vi "HFRR ADV v01.vi"() -> ()   [LabVIEW 2025] (continued)
                frame 81 {
                  n3062 = property on="Air Temperature  ( °C )" class="XYGraph (strict)"("Y Scale.Name Label.Text"=w4075) -> ()  [unwired: 2 in, 2 out]
                }
                frame 82 {
                  n3063 = local write "S 84"(w4076) -> ()
                }
                frame 83 {
                  n3064 = local write "S 85"(w4077) -> ()
                }
                frame 84 {
                  n3065 = local write "S 86"(w4078) -> ()
                }
                frame 85 {
                  n3066 = local write "S 87"(w4079) -> ()
                }
                frame 86 {
                  n3067 = local write "S 88"(w4080) -> ()
                }
                frame 87 {
                  n3068 = property on="FF Calibration g" class="WFGraph (strict)"("Y Scale.Name Label.Text"=w4081) -> ()  [unwired: 2 in, 2 out]
                }
                frame 88 {
                  n3069 = local write "S 90"(w4082) -> ()
                }
                frame 89 {
                  n3070 = local write "S 91"(w4083) -> ()
                }
                frame 90 {
                  n3071 = local write "S 92"(w4084) -> ()
                }
                frame 91 {
                  n3072 = local write "S 93"(w4085) -> ()
                }
                frame 92 {
                  n3073 = local write "S 94"(w4086) -> ()
                }
                frame 93 {
                  n3074 = local write "S 95"(w4087) -> ()
                }
                frame 94 {
                  n3075 = local write "S 96"(w4088) -> ()
                }
                frame 95 {
                  n3076 = local write "S 97"(w4089) -> ()
                }
                frame 96 {
                  n3077 = local write "S 98"(w4090) -> ()
                }
                frame 97 {
                  n3078 = local write "S 99"(w4091) -> ()
                }
                frame 98 {
                  n3079 = local write "S 100"(w4092) -> ()
                }
                frame 99 {
                  n3080 = local write "S 101"(w4093) -> ()
                }
                frame 100 {
                  n3081 = local write "S 102"(w4094) -> ()
                }
                frame 101 {
                  n3082 = local write "S 103"(w4095) -> ()
                }
                frame 102 {
                  n3083 = local write "S 104"(w4096) -> ()
                }
                frame 103 {
                  n3084 = local write "S 105"(w4097) -> ()
                }
                frame 104 {
                  n3085 = local write "S 106"(w4098) -> ()
                }
                frame 105 {
                }
                frame 106 {
                  n3086 = property on="OK Button 17" class="Bool (strict)"("Boolean Text.Text"=w4099) -> ()  [unwired: 2 in, 2 out]
                }
                frame 107 {
                  n3087 = property on="OK Button 16" class="Bool (strict)"("Boolean Text.Text"=w4100) -> ()  [unwired: 2 in, 2 out]
                }
                frame 108 {
                  n3088 = property on="TITTLE" class="Str"("Caption.Text"=w4101) -> ()  [unwired: 2 in, 2 out]
                }
                frame 109 {
                  "String 30" <- w4102
                }
                frame 110 {
                  n3089 = property on="Test Date" class="Str"("Caption.Text"=w4103) -> ()  [unwired: 2 in, 2 out]
                  "String 31" <- w4103
                }
                frame 111 {
                  n3090 = property on="Sample ID" class="Str"("Caption.Text"=w4104) -> ()  [unwired: 2 in, 2 out]
                  "String 32" <- w4104
                }
                frame 112 {
                  n3091 = property on="Tested by" class="Str"("Caption.Text"=w4105) -> ()  [unwired: 2 in, 2 out]
                  "String 33" <- w4105
                }
                frame 113 {
                  n3092 = property on="System Configured Printers 2" class="Arr (strict)"("Caption.Text"=w4106) -> ()  [unwired: 2 in, 2 out]
                }
                frame 114 {
                  n3093 = property on="Selected Printer" class="Str"("Caption.Text"=w4107) -> ()  [unwired: 2 in, 2 out]
                }
                frame 115 {
                  n3094 = property on="Select Printer 3" class="DigNum (strict)"("Caption.Text"=w4108) -> ()  [unwired: 2 in, 2 out]
                }
                frame 116 {
                  n3095 = property on="Print" class="Bool (strict)"("Boolean Text.Text"=w4109) -> ()  [unwired: 2 in, 2 out]
                }
                frame 117 {
                  "String 41" <- w4110
                }
                frame 118 {
                  n3096 = property on="tested by" class="Str"("Caption.Text"=w4111) -> ()  [unwired: 2 in, 2 out]
                }
                frame 119 {
                }
                frame 120 {
                  n3097 = property on="Export" class="Bool (strict)"("Boolean Text.Text"=w4112) -> ()  [unwired: 2 in, 2 out]
                }
                frame 121 {
                  n3098 = property on="TEMP INTERCEPT:" class="DigNum (strict)"("Caption.Text"=w4113) -> ()  [unwired: 2 in, 2 out]
                }
                frame 122 {
                  n3099 = property on="AIR TEMP INTERCEPT:" class="DigNum (strict)"("Caption.Text"=w4114) -> ()  [unwired: 2 in, 2 out]
                }
                frame 123 {
                  n3100 = property on="Select File Type" class="Enum (strict)"("Caption.Text"=w4115) -> ()  [unwired: 2 in, 2 out]
                }
                frame 124 {
                  n3101 = property on="s.NO" class="Str"("Caption.Text"=w4116) -> ()  [unwired: 2 in, 2 out]
                  "String 45" <- w4116
                }
                frame 125 {
                  n3102 = property on="trip1 8" class="Bool (strict)"("Boolean Text.Text"=w4117) -> ()  [unwired: 2 in, 2 out]
                }
                frame 126, Default {
                }
              }
            }
          }
          frame #1 {
            w4125 = TRUE ("Visible")
            n3103 = local read "S 91"() -> (w4142:string)
            n3104 = local read "S 90"() -> (w4141:string)
            n3105 = local read "S 88"() -> (w4140:string)
            n3106 = property on="File Path" class="Path"("Caption.Text"=w4141) -> ()  [unwired: 2 in, 2 out]
            n3107 = property on="SrvM CP" class="Bool (strict)"("Boolean Text.Text"=w4140) -> ()  [unwired: 2 in, 2 out]
            n3108 = local read "S 71"() -> (w4135:string)
            n3109 = local read "S 86"() -> (w4137:string)
            n3110 = local read "S 85"() -> (w4138:string)
            n3111 = local read "S 87"() -> (w4136:string)
            n3112 = local read "S 84"() -> (w4139:string)
            n3113 = local read "S 103"() -> (w4124:string)
            n3114 = local read "S 104"() -> (w4123:string)
            n3115 = property on="ENTER THE NEW PASSWORD" class="Str"("Caption.Text"=w4136) -> ()  [unwired: 2 in, 2 out]
            n3116 = property on="Password" class="Str"("Caption.Text"=w4138) -> ()  [unwired: 2 in, 2 out]
            n3117 = property on="ENTER CURRENT PASSWORD" class="Str"("Caption.Text"=w4137) -> ()  [unwired: 2 in, 2 out]
            n3118 = property on="EDIT" class="Bool (strict)"("Boolean Text.Text"=w4135) -> ()  [unwired: 2 in, 2 out]
            n3119 = property on="SAVE" class="Bool (strict)"("Boolean Text.Text"=w4139) -> ()  [unwired: 2 in, 2 out]
            n3120 = Build Array(w4124, w4123) -> (w4122:string[])
            n3121 = property on="Heater Button" class="Bool (strict)"("Strings [4]"=w4122) -> ()  [unwired: 2 in, 2 out]
            n3122 = property on="CH-HUMIDITY WET" class="DigNum (strict)"("Caption.Size to Text?"=w4125) -> ()  [unwired: 2 in, 2 out]
            n3123 = property on="CH-HUMIDITY DRY" class="DigNum (strict)"("Caption.Size to Text?"=w4125) -> ()  [unwired: 2 in, 2 out]
            n3124 = property on="CH-POWER -" class="DigNum (strict)"("Caption.Size to Text?"=w4125) -> ()  [unwired: 2 in, 2 out]
            n3125 = property on="CH-HEATER" class="DigNum (strict)"("Caption.Size to Text?"=w4125) -> ()  [unwired: 2 in, 2 out]
            n3126 = property on="CH-POWER +" class="DigNum (strict)"("Caption.Size to Text?"=w4125) -> ()  [unwired: 2 in, 2 out]
            n3127 = local read "S 92"() -> (w4134:string)
            n3128 = local read "S 93"() -> (w4133:string)
            n3129 = local read "S 105"() -> (w4120:string)
            n3130 = local read "S 106"() -> (w4119:string)
            n3131 = Build Array(w4134, w4133) -> ()  [unwired: 1 out]
            n3132 = Build Array(w4120, w4119) -> (w4121:string[])
            n3133 = local read "S 95"() -> (w4131:string)
            n3134 = local read "S 94"() -> (w4132:string)
            n3135 = local read "bs"() -> (w4147:string)
            n3136 = local read "as"() -> (w4148:string)
            n3137 = property on="Humidity" class="Bool (strict)"("Strings [4]"=w4121) -> ()  [unwired: 2 in, 2 out]
            n3138 = Concatenate Strings(w4147, "\r", w4148) -> ()  [unwired: 1 out]
            n3139 = property on="STROKE GAIN :" class="DigNum (strict)"("Caption.Text"=w4131) -> ()  [unwired: 2 in, 2 out]
            n3140 = property on="DISPLACEMENT :" class="DigNum (strict)"("Caption.Text"=w4132) -> ()  [unwired: 2 in, 2 out]
            n3141 = property on="Rh After" class="DigNum (strict)"("Caption.Size to Text?"=TRUE ("Caption.Size to Text")) -> ()  [unwired: 2 in, 2 out]
            n3142 = local read "S 48"() -> (w4171:string)
            n3143 = local read "S 50"() -> (w4169:string)
            n3144 = local read "S 51"() -> (w4168:string)
            n3145 = local read "S 49"() -> (w4170:string)
            n3146 = local read "S 52"() -> (w4167:string)
            n3147 = local read "as"() -> (w4152:string)
            n3148 = local read "bs"() -> (w4153:string)
            n3149 = local read "S 56"() -> (w4166:string)
            n3150 = local read "S 57"() -> (w4165:string)
            n3151 = local read "S 58"() -> (w4164:string)
            n3152 = local read "S 59"() -> (w4163:string)
            n3153 = property on="OPEN" class="Bool (strict)"("Boolean Text.Text"=w4167) -> ()  [unwired: 2 in, 2 out]
            n3154 = property on="OPEN 1" class="Bool (strict)"("Boolean Text.Text"=w4171) -> ()  [unwired: 2 in, 2 out]
            n3155 = property on="OPEN 2" class="Bool (strict)"("Boolean Text.Text"=w4170) -> ()  [unwired: 2 in, 2 out]
            n3156 = property on="OPEN 3" class="Bool (strict)"("Boolean Text.Text"=w4169) -> ()  [unwired: 2 in, 2 out]
            n3157 = property on="OPEN 4" class="Bool (strict)"("Boolean Text.Text"=w4168) -> ()  [unwired: 2 in, 2 out]
            n3158 = Concatenate Strings(w4153, "\r", w4152) -> ()  [unwired: 1 out]
            n3159 = local read "S 102"() -> (w4126:string)
            n3160 = property on="КОФ1" class="DigNum (strict)"("Caption.Text"=w4166) -> ()  [unwired: 2 in, 2 out]
            n3161 = local read "S 98"() -> (w4130:string)
            n3162 = local read "S 99"() -> (w4129:string)
            n3163 = local read "S 100"() -> (w4128:string)
            n3164 = local read "S 101"() -> (w4127:string)
            n3165 = property on="КОФ2" class="DigNum (strict)"("Caption.Text"=w4165) -> ()  [unwired: 2 in, 2 out]
            n3166 = property on="КОФ3" class="DigNum (strict)"("Caption.Text"=w4164) -> ()  [unwired: 2 in, 2 out]
            n3167 = property on="КОФ4" class="DigNum (strict)"("Caption.Text"=w4163) -> ()  [unwired: 2 in, 2 out]
            n3168 = local read "bs"() -> (w4151:string)
            n3169 = local read "as"() -> (w4150:string)
            n3170 = property on="CH-POWER +" class="DigNum (strict)"("Caption.Text"=w4130) -> ()  [unwired: 2 in, 2 out]
            n3171 = property on="CH-POWER -" class="DigNum (strict)"("Caption.Text"=w4129) -> ()  [unwired: 2 in, 2 out]
            n3172 = property on="CH-HEATER" class="DigNum (strict)"("Caption.Text"=w4128) -> ()  [unwired: 2 in, 2 out]
            n3173 = property on="CH-HUMIDITY DRY" class="DigNum (strict)"("Caption.Text"=w4127) -> ()  [unwired: 2 in, 2 out]
            n3174 = property on="CH-HUMIDITY WET" class="DigNum (strict)"("Caption.Text"=w4126) -> ()  [unwired: 2 in, 2 out]
            n3175 = local read "S 60"() -> (w4162:string)
            n3176 = local read "S 54"() -> (w4172:string)
            n3177 = Concatenate Strings(w4151, "\r", w4150) -> ()  [unwired: 1 out]
            n3178 = Concatenate Strings(w4172, w4162) -> ()  [unwired: 1 out]
            n3179 = local read "S 77"() -> (→"String 43":string)
            n3180 = local read "S 76"() -> (w4145:string)
            n3181 = local read "S 78"() -> (w4144:string)
            n3182 = local read "S 71"() -> (w4156:string)
            n3183 = local read "S 66"() -> (w4161:string)
            n3184 = local read "S 67"() -> (w4160:string)
            n3185 = local read "S 68"() -> (w4159:string)
            n3186 = local read "S 69"() -> (w4158:string)
            n3187 = local read "S 70"() -> (w4157:string)
            n3188 = property on="AIR TEMP" class="DigNum (strict)"("Caption.Text"=w4144) -> ()  [unwired: 2 in, 2 out]
            n3189 = property on="Set Strk" class="DigNum (strict)"("Caption.Text"=w4145) -> ()  [unwired: 2 in, 2 out]
            n3190 = property on="FRIC. FORCE :" class="DigNum (strict)"("Caption.Text"=w4161) -> ()  [unwired: 2 in, 2 out]
            n3191 = property on="TEMPERATURE :" class="DigNum (strict)"("Caption.Text"=w4160) -> ()  [unwired: 2 in, 2 out]
            n3192 = property on="SPEED OUT:" class="DigNum (strict)"("Caption.Text"=w4159) -> ()  [unwired: 2 in, 2 out]
            n3193 = property on="AIR TEMPERATURE :" class="DigNum (strict)"("Caption.Text"=w4158) -> ()  [unwired: 2 in, 2 out]
            n3194 = property on="HUMIDITY:" class="DigNum (strict)"("Caption.Text"=w4157) -> ()  [unwired: 2 in, 2 out]
            n3195 = property on="EDIT" class="Bool (strict)"("Boolean Text.Text"=w4156) -> ()  [unwired: 2 in, 2 out]
            n3196 = local read "S 79"() -> (w4143:string)
          }
          frame #2 {
          }
        }
        n3197 = local write "Lan flag"(10.0 ("Lan flag")) -> ()
      }
      frame Enabled {
      }
    }
    n3198 = Wait (ms)(milliseconds to wait=u32 2000) -> ()  [unwired: 1 out]
    n3199 = local read "Quit"() -> (w3945:bool)
  }
  n3200 = disable-structure shown="Disabled" {
    frame Disabled {
      n3201 = while {
        tunnel: [w4174] -> _
        i -> [w4174]
        stop <- w4173 continue-if-true
        n3202 = Wait (ms)(milliseconds to wait=u32 50) -> ()  [unwired: 1 out]
        n3203 = stacked-sequence {
          frame #0 {
            # "Controls Text color"
            # "Controls BG color"
            n3204 = property on="FILE" class="Str"("Text.Text Colors:Text Color"="SC  Text") -> ()  [unwired: 2 in, 2 out]
            n3205 = property on="Fuel Discription :" class="Str"("Text.Text Colors:Text Color"="SC  Text") -> ()  [unwired: 2 in, 2 out]
            n3206 = property on="tested by" class="Str"("Text.Text Colors:Text Color"="SC  Text") -> ()  [unwired: 2 in, 2 out]
            n3207 = property on="Remarks :" class="Str"("Text.Text Colors:Text Color"="SC  Text") -> ()  [unwired: 2 in, 2 out]
            n3208 = property class="DigNum (strict)"("Numeric Text.Text Colors:BG Color"="NC BG") -> ()  [unwired: 2 in, 2 out]
            n3209 = property class="DigNum (strict)"("Numeric Text.Text Colors:BG Color"="NC BG") -> ()  [unwired: 2 in, 2 out]
            n3210 = property class="DigNum (strict)"("Numeric Text.Text Colors:BG Color"="NC BG") -> ()  [unwired: 2 in, 2 out]
            n3211 = property class="DigNum (strict)"("Numeric Text.Text Colors:BG Color"="NC BG") -> ()  [unwired: 2 in, 2 out]
            n3212 = property class="DigNum (strict)"("Numeric Text.Text Colors:BG Color"="NC BG") -> ()  [unwired: 2 in, 2 out]
            n3213 = property class="DigNum (strict)"("Numeric Text.Text Colors:BG Color"="NC BG") -> ()  [unwired: 2 in, 2 out]
            n3214 = property class="DigNum (strict)"("Numeric Text.Text Colors:BG Color"="NC BG") -> ()  [unwired: 2 in, 2 out]
            n3215 = property class="DigNum (strict)"("Numeric Text.Text Colors:BG Color"="NC BG") -> ()  [unwired: 2 in, 2 out]
            n3216 = property class="DigNum (strict)"("Numeric Text.Text Colors:BG Color"="NC BG") -> ()  [unwired: 2 in, 2 out]
            n3217 = property class="DigNum (strict)"("Numeric Text.Text Colors:BG Color"="NC BG") -> ()  [unwired: 2 in, 2 out]
            n3218 = property class="DigNum (strict)"("Numeric Text.Text Colors:BG Color"="NC BG") -> ()  [unwired: 2 in, 2 out]
            n3219 = property class="DigNum (strict)"("Numeric Text.Text Colors:BG Color"="NC BG") -> ()  [unwired: 2 in, 2 out]
            n3220 = property on="FILE" class="Str"("Text.Text Colors:BG Color"="SC BG 3") -> ()  [unwired: 2 in, 2 out]
            n3221 = property on="Fuel Discription :" class="Str"("Text.Text Colors:BG Color"="SC BG 3") -> ()  [unwired: 2 in, 2 out]
            n3222 = property on="tested by" class="Str"("Text.Text Colors:BG Color"="SC BG 3") -> ()  [unwired: 2 in, 2 out]
            n3223 = property on="Remarks :" class="Str"("Text.Text Colors:BG Color"="SC BG 3") -> ()  [unwired: 2 in, 2 out]
            n3224 = property class="DigNum (strict)"("Numeric Text.Text Colors:Text Color"="NC Text") -> ()  [unwired: 2 in, 2 out]
            n3225 = property class="DigNum (strict)"("Numeric Text.Text Colors:Text Color"="NC Text") -> ()  [unwired: 2 in, 2 out]
            n3226 = property class="DigNum (strict)"("Numeric Text.Text Colors:Text Color"="NC Text") -> ()  [unwired: 2 in, 2 out]
            n3227 = property class="DigNum (strict)"("Numeric Text.Text Colors:Text Color"="NC Text") -> ()  [unwired: 2 in, 2 out]
            n3228 = property class="DigNum (strict)"("Numeric Text.Text Colors:Text Color"="NC Text") -> ()  [unwired: 2 in, 2 out]
            n3229 = property class="DigNum (strict)"("Numeric Text.Text Colors:Text Color"="NC Text") -> ()  [unwired: 2 in, 2 out]
            n3230 = property class="DigNum (strict)"("Numeric Text.Text Colors:Text Color"="NC Text") -> ()  [unwired: 2 in, 2 out]
            n3231 = property class="DigNum (strict)"("Numeric Text.Text Colors:Text Color"="NC Text") -> ()  [unwired: 2 in, 2 out]
            n3232 = property class="DigNum (strict)"("Numeric Text.Text Colors:Text Color"="NC Text") -> ()  [unwired: 2 in, 2 out]
            n3233 = property class="DigNum (strict)"("Numeric Text.Text Colors:Text Color"="NC Text") -> ()  [unwired: 2 in, 2 out]
            n3234 = property class="DigNum (strict)"("Numeric Text.Text Colors:Text Color"="NC Text") -> ()  [unwired: 2 in, 2 out]
            n3235 = property class="DigNum (strict)"("Numeric Text.Text Colors:Text Color"="NC Text") -> ()  [unwired: 2 in, 2 out]
            n3236 = property class="DigNum (strict)"("Numeric Text.Text Colors:Text Color"="NI Text  2") -> ()  [unwired: 2 in, 2 out]
            n3237 = property class="DigNum (strict)"("Numeric Text.Text Colors:Text Color"="NI Text  2") -> ()  [unwired: 2 in, 2 out]
            n3238 = property class="DigNum (strict)"("Numeric Text.Text Colors:Text Color"="NI Text  2") -> ()  [unwired: 2 in, 2 out]
            n3239 = property class="DigNum (strict)"("Numeric Text.Text Colors:Text Color"="NI Text  2") -> ()  [unwired: 2 in, 2 out]
            n3240 = property class="DigNum (strict)"("Numeric Text.Text Colors:Text Color"="NI Text  2") -> ()  [unwired: 2 in, 2 out]
            n3241 = property class="DigNum (strict)"("Numeric Text.Text Colors:Text Color"="NI Text  2") -> ()  [unwired: 2 in, 2 out]
            n3242 = property class="DigNum (strict)"("Numeric Text.Text Colors:Text Color"="NI Text  2") -> ()  [unwired: 2 in, 2 out]
            n3243 = property class="DigNum (strict)"("Numeric Text.Text Colors:Text Color"="NI Text  2") -> ()  [unwired: 2 in, 2 out]
            n3244 = property class="DigNum (strict)"("Numeric Text.Text Colors:Text Color"="NI Text  2") -> ()  [unwired: 2 in, 2 out]
            n3245 = property class="DigNum (strict)"("Numeric Text.Text Colors:Text Color"="NI Text  2") -> ()  [unwired: 2 in, 2 out]
            n3246 = property class="DigNum (strict)"("Numeric Text.Text Colors:Text Color"="NI Text  2") -> ()  [unwired: 2 in, 2 out]
            n3247 = property class="DigNum (strict)"("Numeric Text.Text Colors:Text Color"="NI Text  2") -> ()  [unwired: 2 in, 2 out]
            n3248 = property class="DigNum (strict)"("Numeric Text.Text Colors:Text Color"="NI Text  2") -> ()  [unwired: 2 in, 2 out]
            n3249 = property class="DigNum (strict)"("Numeric Text.Text Colors:Text Color"="NI Text  2") -> ()  [unwired: 2 in, 2 out]
            n3250 = property class="DigNum (strict)"("Numeric Text.Text Colors:Text Color"="NI Text  2") -> ()  [unwired: 2 in, 2 out]
            n3251 = property on="Coefficient Of Friction" class="XYGraph (strict)"("Plot Area:Colors:FG Color"="GFG  2", "Plot Area:Colors:BG Color"="GBG   2") -> ()  [unwired: 2 in, 2 out]
            n3252 = property on="Humidity ( %RH )" class="XYGraph (strict)"("Plot Area:Colors:FG Color"="GFG  2", "Plot Area:Colors:BG Color"="GBG   2") -> ()  [unwired: 2 in, 2 out]
            n3253 = property on="Air Temperature  ( °C )" class="XYGraph (strict)"("Plot Area:Colors:FG Color"="GFG  2", "Plot Area:Colors:BG Color"="GBG   2") -> ()  [unwired: 2 in, 2 out]
            n3254 = property on="Sample Temperature ( °C )" class="XYGraph (strict)"("Plot Area:Colors:FG Color"="GFG  2", "Plot Area:Colors:BG Color"="GBG   2") -> ()  [unwired: 2 in, 2 out]
            n3255 = property class="DigNum (strict)"("Numeric Text.Text Colors:BG Color"="NI BG 2") -> ()  [unwired: 2 in, 2 out]
            n3256 = property class="DigNum (strict)"("Numeric Text.Text Colors:BG Color"="NI BG 2") -> ()  [unwired: 2 in, 2 out]
            n3257 = property class="DigNum (strict)"("Numeric Text.Text Colors:BG Color"="NI BG 2") -> ()  [unwired: 2 in, 2 out]
            n3258 = property class="DigNum (strict)"("Numeric Text.Text Colors:BG Color"="NI BG 2") -> ()  [unwired: 2 in, 2 out]
            n3259 = property class="DigNum (strict)"("Numeric Text.Text Colors:BG Color"="NI BG 2") -> ()  [unwired: 2 in, 2 out]
            n3260 = property class="DigNum (strict)"("Numeric Text.Text Colors:BG Color"="NI BG 2") -> ()  [unwired: 2 in, 2 out]
            n3261 = property class="DigNum (strict)"("Numeric Text.Text Colors:BG Color"="NI BG 2") -> ()  [unwired: 2 in, 2 out]
            n3262 = property class="DigNum (strict)"("Numeric Text.Text Colors:BG Color"="NI BG 2") -> ()  [unwired: 2 in, 2 out]
            n3263 = property class="DigNum (strict)"("Numeric Text.Text Colors:BG Color"="NI BG 2") -> ()  [unwired: 2 in, 2 out]
            n3264 = property class="DigNum (strict)"("Numeric Text.Text Colors:BG Color"="NI BG 2") -> ()  [unwired: 2 in, 2 out]
            n3265 = property class="DigNum (strict)"("Numeric Text.Text Colors:BG Color"="NI BG 2") -> ()  [unwired: 2 in, 2 out]
            n3266 = property class="DigNum (strict)"("Numeric Text.Text Colors:BG Color"="NI BG 2") -> ()  [unwired: 2 in, 2 out]
            n3267 = property class="DigNum (strict)"("Numeric Text.Text Colors:BG Color"="NI BG 2") -> ()  [unwired: 2 in, 2 out]
            n3268 = property class="DigNum (strict)"("Numeric Text.Text Colors:BG Color"="NI BG 2") -> ()  [unwired: 2 in, 2 out]
            n3269 = property class="DigNum (strict)"("Numeric Text.Text Colors:BG Color"="NI BG 2") -> ()  [unwired: 2 in, 2 out]
            n3270 = property class="Bool"("Colors [4]"="Boolean BC T & BG") -> ()  [unwired: 2 in, 2 out]
            n3271 = property on="Save & Continue" class="Bool (strict)"("Colors [4]"="Boolean BC T & BG") -> ()  [unwired: 2 in, 2 out]
            n3272 = property on="Heater Button" class="Bool (strict)"("Colors [4]"="Boolean BC T & BG") -> ()  [unwired: 2 in, 2 out]
            n3273 = property class="Bool"("Colors [4]"="Boolean BC T & BG") -> ()  [unwired: 2 in, 2 out]
            n3274 = property on="Humidity" class="Bool (strict)"("Colors [4]"="Boolean BC T & BG") -> ()  [unwired: 2 in, 2 out]
            n3275 = property class="Bool (strict)"("Colors [4]"="Boolean BC T & BG") -> ()  [unwired: 2 in, 2 out]
            n3276 = property on="RUN" class="Bool (strict)"("Colors [4]"="Boolean BC T & BG") -> ()  [unwired: 2 in, 2 out]
            n3277 = property on="trip1 8" class="Bool (strict)"("Colors [4]"="Boolean BC T & BG") -> ()  [unwired: 2 in, 2 out]
            n3278 = property class="Bool"("Colors [4]"="Boolean BC T & BG") -> ()  [unwired: 2 in, 2 out]
            n3279 = property class="Bool (strict)"("Colors [4]"="Boolean BC T & BG") -> ()  [unwired: 2 in, 2 out]
            n3280 = property on="OPEN 1" class="Bool (strict)"("Colors [4]"="Boolean BC T & BG 2") -> ()  [unwired: 2 in, 2 out]
            n3281 = property on="OPEN 2" class="Bool (strict)"("Colors [4]"="Boolean BC T & BG 2") -> ()  [unwired: 2 in, 2 out]
            n3282 = property on="OPEN 3" class="Bool (strict)"("Colors [4]"="Boolean BC T & BG 2") -> ()  [unwired: 2 in, 2 out]
            n3283 = property on="OPEN 4" class="Bool (strict)"("Colors [4]"="Boolean BC T & BG 2") -> ()  [unwired: 2 in, 2 out]
            n3284 = property on="OPEN" class="Bool (strict)"("Colors [4]"="Boolean BC T & BG 2") -> ()  [unwired: 2 in, 2 out]
            n3285 = property on="rstv2" class="Bool"("Colors [4]"="Boolean BC T & BG 2") -> ()  [unwired: 2 in, 2 out]
            n3286 = property on="RST CP" class="Bool"("Colors [4]"="Boolean BC T & BG 2") -> ()  [unwired: 2 in, 2 out]
            n3287 = property on="RSTV1 3" class="Bool"("Colors [4]"="Boolean BC T & BG 2") -> ()  [unwired: 2 in, 2 out]
            n3288 = property on="RSTV1 2" class="Bool"("Colors [4]"="Boolean BC T & BG 2") -> ()  [unwired: 2 in, 2 out]
          }
          frame #1 {
          }
        }
        n3289 = local read "Quit"() -> (w4173:bool)
      }
    }
    frame Enabled {
    }
  }
  n3290 = while {
    shift-right: [w4191] -> _
    shift-left: _ -> [w4192]
    shift-right: [w4189] -> _
    shift-left: T16 {"Read Heave and Surge"="", "Bytes at Heave Port"=0.0, "Heave and Surge COM Port:"="COM9", "Com Port 2"="COM7", "Residual Due"="", "Heave COM Status 2"=TRUE, "Heave COM Status"=TRUE, "Port 2"=TRUE, "Sway PPR"=6400.0, "Surge PPR"=6400.0, "Heave PPR"=6400.0, "Sway Pitch"=2.0, "Surge Pitch"=3.0, "Heave Pitch"=4.0, "Sway Pulses/mm"=320.0, "Surge Pulses/mm"=1600.0, "Heave Pulses/mm"=1600.0, "inner loop"=0.0, "Read Heave and Surge 2"="", "String 36"="", "Write S"=FALSE, "WriteCC1"=[""], "Heave COM Loop"=0, "LastCom"="", "EXIT"=FALSE, "Error Heave"={"status"=TRUE, "code"=-1073807343, "source"=""}} -> [w4188]
    shift-right: [w4186] -> _
    shift-left: enum16{"init", "MAIN", "Panel Close"}."init" -> [w4187]
    stop <- w4190 stop-if-true
    n3291 = case shown="\"init\"" w4187 {
      tunnel: w4192 -> [w4206 w4221 w4291 w4293]
      tunnel: [w4200 w4239 w4291 w4293] -> w4191
      tunnel: [_ _ TRUE _] -> w4190
      tunnel: [w4196 w4236 w4289 w4292] -> w4189
      tunnel: w4188 -> [w4203 w4220 w4289 w4292]
      tunnel: [enum16{"init", "MAIN", "Panel Close"}."MAIN" w4214 _ _] -> w4186
      frame "init" {
        n3292 = Bundle By Name(cluster=w4203, "Heave and Surge COM Port:"="C3 :") -> (w4202:T16)
        n3293 = call "Instrument fgv.vi"("Enum"=T26."INIT", "error in (no error) 2"=w4206, "INPUT"=w4202) -> ("error"=w4204:errorcluster, "output"=w4199:T16)  [unwired: 6 in, 1 out]
        n3294 = case shown="No Error" w4204 {
          selector: w4204 -> [w4208 _]
          tunnel: [w4208 w4212] -> w4200
          tunnel: w4199 -> [w4207 w4210]
          tunnel: [w4207 w4209] -> w4197
          frame No Error {
          }
          frame Error {
            n3295 = call "Instrument fgv.vi"("Enum"=T26."ERROR INIT", "INPUT"=w4210) -> ("error"=w4213:errorcluster, "output"=w4209:T16)  [unwired: 7 in, 1 out]
            n3296 = call <vilib>:"Clear Errors.vi"("error in (no error)"=w4213) -> ("error out"=w4212:errorcluster)  [unwired: 5 in, 1 out]
          }
        }
        n3297 = local read "LastCom"() -> (w4195:string)
        n3298 = Unbundle By Name(w4197) -> ("Heave COM Status 2"=→"COM Status" →"Instrument Status":bool, "Error Heave"=→"Error":errorcluster)  [unwired: 1 out]
        n3299 = Bundle By Name(cluster=w4197, "LastCom"=w4195) -> (w4196:T16)
      }
      frame "MAIN" {
        n3300 = Unbundle By Name(w4220) -> ("Com Port 2"=w4241:refnum<visa-resource-name>)
        n3301 = local write "Com Port 4"(w4241) -> ()
        n3302 = local read "C3 :"() -> (w4218:refnum<visa-resource-name>)
        n3303 = Divide(x="Heave PPR", y="Heave Pitch") -> (x/y=→"Heave Pulses/mm":dbl)
        n3304 = Bundle By Name(cluster=w4220, "Heave and Surge COM Port:"=w4218) -> (w4219:T16)
        n3305 = Equal?(x=w4241, y=w4218) -> (x = y?=w4240:bool)
        n3306 = Divide(x="Sway PPR", y="Sway Pitch") -> (x/y=→"Sway Pulses/mm":dbl)
        n3307 = case shown="False" w4240 {
          tunnel: [w4245 w4262] -> w4239
          tunnel: w4221 -> [w4246 w4268]
          tunnel: w4219 -> [w4244 w4266]
          tunnel: [w4243 w4261] -> w4236
          frame False {
            n3308 = call <vilib>:"Clear Errors.vi"("error in (no error)"=w4246) -> ("error out"=w4242:errorcluster)  [unwired: 5 in, 1 out]
            n3309 = call "Instrument fgv.vi"("Enum"=T26."ERROR INIT", "error in (no error) 2"=w4242, "INPUT"=w4244) -> ("error"=w4248:errorcluster, "output"=w4243:T16)  [unwired: 6 in, 1 out]
            n3310 = call <vilib>:"Clear Errors.vi"("error in (no error)"=w4248) -> ("error out"=w4245:errorcluster)  [unwired: 5 in, 1 out]
          }
          frame True {
            n3311 = call "Instrument fgv.vi"("Enum"=T26."READ", "error in (no error) 2"=w4268, "INPUT"=w4266) -> ("error"=w4267:errorcluster, "output"=w4258:T16)  [unwired: 6 in, 1 out]
            n3312 = Bundle By Name(cluster=w4258, "String 36"="String 11") -> (w4257:T16)
            n3313 = case shown="True" "Write S" {
              selector: "Write S" -> [_ w4288]
              tunnel: w4267 -> [w4281 w4287]
              tunnel: [w4281 w4286] -> w4254
              tunnel: w4257 -> [w4280 w4283]
              tunnel: [w4280 w4282] -> w4253
              frame False {
              }
              frame True {
                n3314 = Not(x=w4288) -> (.not. x?=w4284:bool)
                n3315 = local write "Write S"(w4284) -> ()
                n3316 = call "Instrument fgv.vi"("Enum"=T26."MANUAL WRITE", "error in (no error) 2"=w4287, "INPUT"=w4283) -> ("error"=w4286:errorcluster, "output"=w4282:T16)  [unwired: 6 in, 1 out]
              }
            }
            n3317 = Array Size(array="WriteHumidity") -> (size(s)=w4251:i32)
            n3318 = Greater Than 0?(x=w4251) -> (x > 0?=w4249:bool)
            n3319 = call "Instrument fgv.vi"("Enum"=T26."WRITE", "error in (no error) 2"=w4254, "WriteCC1"="WriteHumidity", "INPUT"=w4253) -> ("error"=w4264:errorcluster, "WriteCC1 2"=w4252:string[], "output"=w4263:T16)  [unwired: 5 in]
            n3320 = case shown="True" w4249 {
              tunnel: w4252 -> [_ w4270]
              frame False {
              }
              frame True {
                n3321 = local write "WriteHumidity"(w4270) -> ()
              }
            }
            n3322 = case shown="Error" w4264 {
              selector: w4264 -> [w4271 w4274]
              tunnel: w4263 -> [w4272 w4279]
              tunnel: [w4272 w4278] -> w4261
              tunnel: [w4271 w4276] -> w4262
              frame No Error {
              }
              frame Error {
                n3323 = call <vilib>:"Clear Errors.vi"("error in (no error)"=w4274) -> ("error out"=w4273:errorcluster)  [unwired: 5 in, 1 out]
                n3324 = call "Instrument fgv.vi"("Enum"=T26."ERROR INIT", "error in (no error) 2"=w4273, "INPUT"=w4279) -> ("error"=w4277:errorcluster, "output"=w4278:T16)  [unwired: 6 in, 1 out]
                n3325 = call <vilib>:"Clear Errors.vi"("error in (no error)"=w4277) -> ("error out"=w4276:errorcluster)  [unwired: 5 in, 1 out]
              }
            }
            n3326 = Unbundle By Name(w4261) -> ("LastCom"=→"LastCom":string, "Read Heave and Surge"=→"Read Humidity":string)
          }
        }
        n3327 = Divide(x="Surge PPR", y="Surge Pitch") -> (x/y=→"Surge Pulses/mm":dbl)
        n3328 = Unbundle By Name(w4236) -> ("Heave COM Status 2"=w4238:bool, "Heave COM Status"=w4237:bool, "Error Heave"=w4234:errorcluster, "Bytes at Heave Port"=→"Bytes at Humidity Port":dbl)
        n3329 = Unbundle By Name(w4234) -> ("status"=→"Humidity Port":bool)
        n3330 = Not(x=w4237) -> (.not. x?=w4222:bool)
        n3331 = local write "Error"(w4234) -> ()
        n3332 = Not(x=w4238) -> (.not. x?=w4223:bool)
        n3333 = local write "Instrument Status"(w4222) -> ()
        n3334 = local write "COM Status"(w4223) -> ()
        n3335 = local read "Quit"() -> (w4215:bool)
        n3336 = Select(t=enum16{"init", "MAIN", "Panel Close"}."Panel Close", s=w4215, f=enum16{"init", "MAIN", "Panel Close"}."MAIN") -> (s? t:f=w4214:enum16{"init", "MAIN", "Panel Close"})
      }
      frame "Panel Close" {
      }
      frame Default {
      }
    }
  }
  n3337 = while {
    stop <- w4319 stop-if-true
    n3338 = local read "Read Humidity"() -> (w4300:string)
    n3339 = call <vilib>:"High Resolution Polling Wait.vi"("seconds to wait"=0.1) -> ()  [unwired: 10 in, 1 out]
    n3340 = Spreadsheet String To Array(delimiter (Tab)=",", format string="", spreadsheet string=w4300, array type (2D Dbl)=string[] []) -> (array=w4314:string[])
    n3341 = for {
      tunnel: w4314 -> [w4324] mode=indexing
      tunnel: string[] ["STATE;", "SET;", "RH;", "T;", "AMB_RH;", "AMB_T;", "PUMP;", "FAN_IN;", "FAN_OUT;", "DEHUM;", "CURRENT;", "STALL;"] -> [w4323] mode=indexing
      tunnel: [w4322] -> w4313 mode=indexing
      n3342 = Match Pattern(string=w4324, regular expression=w4323) -> (after substring=w4322:string)  [unwired: 1 in, 3 out]
    }
    n3343 = Index Array(array=w4313) -> (element #1=→"STATE :":string, element #2=→"SET :":string, element #3=w4302:string, element #4=→"T :":string, element #5=w4299:string, element #6=→"AMB_T :":string, element #7=→"PUMP :":string, element #8=→"FAN_IN :":string, element #9=→"FAN_OUT :":string, element #10=→"DEHUM :":string, element #11=→"CURRENT :":string, element #12=→"STALL :":string)  [unwired: 12 in]
    "RH :" <- w4302
    "AMB_RH :" <- w4299
    n3344 = Fract/Exp String To Number(string=w4302) -> (number=w4294:dbl)  [unwired: 3 in, 1 out]
    n3345 = Fract/Exp String To Number(string=w4299) -> (number=w4298:dbl)  [unwired: 3 in, 1 out]
    n3346 = local write "Ambient Humidity :"(w4298) -> ()
    n3347 = Equal?(x=w4294, y=0.0) -> (x = y?=w4296:bool)
    n3348 = case shown="True" w4296 {
      tunnel: [w4320 w4321] -> w4295
      tunnel: w4294 -> [w4320 _]
      frame False {
        (unwired) 0.0
        "Humidity temp" <- w4320
      }
      frame True {
        n3349 = local read "Humidity temp"() -> (w4321:dbl)
      }
    }
    "RH Numeric:" <- w4295
    n3350 = local read "Quit"() -> (w4319:bool)
  }
  n3351 = disable-structure shown="Disabled" {
    frame Disabled {
      n3352 = while {
        tunnel: [w4558] -> _
        i -> [w4558]
        stop <- w4555 stop-if-true
        n3353 = local read "powstat"() -> (w4556:bool)
        n3354 = case shown="True" w4556 {
          frame False {
          }
          frame True {
            n3355 = local read "RUN"() -> (w4559:bool)
            n3356 = case shown="True" w4559 {
              frame False {
                w4589 = 65.0 ("y")
                n3357 = local read "Set Hz"() -> (w4617:dbl)
                n3358 = local read "NORMAL LOAD"() -> (w4618:dbl)
                n3359 = Multiply(x=w4617, y=60.0) -> (x*y=w4624:dbl)
                n3360 = Multiply(x=1.2 ("y"), y=0.949) -> (x*y=w4593:dbl)
                n3361 = Multiply(x=1.2 ("y"), y=0.8166) -> (x*y=w4597:dbl)
                n3362 = Multiply(x=1.2 ("y"), y=0.851) -> (x*y=w4592:dbl)
                n3363 = local read "FF 2"() -> (w4616:dbl)
                n3364 = Absolute Value(x=w4624) -> (abs(x)=w4622:dbl)
                n3365 = case shown="13.." w4616 {
                  tunnel: [1 2 3] -> w4614
                  frame 0..10, Default {
                    # "Normal"
                  }
                  frame 11, 12 {
                  }
                  frame 13.. {
                  }
                }
                "FF STATE" <- w4614
                n3366 = local read "TEMP"() -> (w4577:dbl)
                n3367 = local read item#-1() -> (w4591)
                n3368 = Less?(x=w4591, y=w4597) -> (x < y?=w4594:bool)
                n3369 = In Range and Coerce(upper limit=w4593, x=w4591, lower limit=w4592) -> (In Range?=w4595:bool)  [unwired: 1 out]
                n3370 = case shown="3601.." w4622 {
                  tunnel: [1 2 3] -> w4620
                  frame 0..3000, Default {
                    # "Normal"
                  }
                  frame 3001..3600 {
                  }
                  frame 3601.. {
                  }
                }
                n3371 = case shown="11.." w4618 {
                  tunnel: [1 3] -> w4619
                  frame 1..10, Default {
                  }
                  frame 11.. {
                  }
                }
                "NL STATE" <- w4619
                n3372 = Multiply(x=1.2 ("y"), y=0.95) -> (x*y=w4607:dbl)
                n3373 = Multiply(x=w4589, y=0.954) -> (x*y=w4581:dbl)
                n3374 = Or(x=w4594, y=w4595) -> (x .or. y?=w4596:bool)
                n3375 = Greater Or Equal?(x=w4591, y=w4607) -> (x >= y?=w4604:bool)
                n3376 = Multiply(x=w4589, y=0.99) -> (x*y=w4578:dbl)
                n3377 = Greater Or Equal?(x=w4577, y=w4578) -> (x >= y?=w4583:bool)
                n3378 = Greater Or Equal?(x=w4577, y=w4581) -> (x >= y?=w4580:bool)
                n3379 = case shown="0, 1, Default" w4591 {
                  tunnel: [1 3] -> w4608
                  frame 0, 1, Default {
                  }
                  frame 2.. {
                  }
                }
                n3380 = case shown="True" w4604 {
                  tunnel: [1 3] -> w4609
                  frame False {
                  }
                  frame True {
                  }
                }
                n3381 = case shown="True" w4596 {
                  tunnel: [1 2] -> w4610
                  frame False {
                  }
                  frame True {
                  }
                }
                n3382 = case shown="..0" w4577 {
                  tunnel: [2 3 3 1] -> w4584
                  frame 61, 62 {
                  }
                  frame 63.. {
                  }
                  frame ..0 {
                  }
                  frame 10..60, Default {
                  }
                }
                n3383 = case shown="True" w4583 {
                  tunnel: [1 3] -> w4585
                  frame False {
                  }
                  frame True {
                  }
                }
                n3384 = Number To Decimal String(number=w4620) -> (decimal integer string=w4621:string)  [unwired: 1 in]
                n3385 = case shown="True" w4580 {
                  tunnel: [1 2] -> w4586
                  frame False {
                  }
                  frame True {
                  }
                }
                n3386 = Number To Decimal String(number=1) -> (decimal integer string=→"Air temp":string)  [unwired: 1 in]
                n3387 = Number To Decimal String(number=w4614) -> (decimal integer string=→"ff_st":string)  [unwired: 1 in]
                n3388 = local write "sp_st"(w4621) -> ()
                n3389 = Number To Decimal String(number=w4619) -> (decimal integer string=→"nl_st":string)  [unwired: 1 in]
                n3390 = Build Array(w4584, w4585, w4586) -> (w4587:i32[])
                n3391 = Build Array(w4608, w4609, w4610) -> (w4611:i32[])
                n3392 = Array Max & Min(array=w4587) -> (max value=w4588:i32)  [unwired: 3 out]
                n3393 = Array Max & Min(array=w4611) -> (max value=w4612:i32)  [unwired: 3 out]
                n3394 = Number To Decimal String(number=w4588) -> (decimal integer string=w4576:string)  [unwired: 1 in]
                n3395 = Number To Decimal String(number=w4612) -> (decimal integer string=→"Stroke Ln 2":string)  [unwired: 1 in]
                n3396 = local write "temp_st"(w4576) -> ()
              }
              frame True {
                w4674 = 65.0 ("y")
                # "Healthy -1\nWarning -2\nError -3"
                n3397 = local read "TEMP"() -> (w4685:dbl)
                n3398 = local read "NORMAL LOAD"() -> (w4689:dbl)
                n3399 = local read "Set Hz"() -> (w4687:dbl)
                n3400 = Multiply(x=1.2 ("y"), y=0.949) -> (x*y=w4669:dbl)
                n3401 = Multiply(x=1.2 ("y"), y=0.8166) -> (x*y=w4665:dbl)
                n3402 = Multiply(x=1.2 ("y"), y=0.851) -> (x*y=w4670:dbl)
                n3403 = Multiply(x=w4674, y=0.954) -> (x*y=w4681:dbl)
                n3404 = Multiply(x=w4674, y=0.99) -> (x*y=w4684:dbl)
                n3405 = Greater Or Equal?(x=w4685, y=w4684) -> (x >= y?=w4679:bool)
                n3406 = Multiply(x=w4687, y=60.0) -> (x*y=w4693:dbl)
                n3407 = Greater Or Equal?(x=w4685, y=w4681) -> (x >= y?=w4682:bool)
                n3408 = local read "FF 2"() -> (w4688:dbl)
                n3409 = local read item#-1() -> (w4671)
                n3410 = Less?(x=w4671, y=w4665) -> (x < y?=w4668:bool)
                n3411 = In Range and Coerce(upper limit=w4669, x=w4671, lower limit=w4670) -> (In Range?=w4667:bool)  [unwired: 1 out]
                n3412 = Absolute Value(x=w4693) -> (abs(x)=w4691:dbl)
                n3413 = case shown="63.." w4685 {
                  tunnel: [2 3 3 1] -> w4678
                  frame 61, 62 {
                  }
                  frame 63.. {
                  }
                  frame ..0 {
                  }
                  frame 10..60, Default {
                  }
                }
                n3414 = case shown="True" w4679 {
                  tunnel: [1 3] -> w4677
                  frame False {
                  }
                  frame True {
                  }
                }
                n3415 = case shown="True" w4682 {
                  tunnel: [1 2] -> w4676
                  frame False {
                  }
                  frame True {
                  }
                }
                n3416 = Multiply(x=1.2 ("y"), y=0.95) -> (x*y=w4655:dbl)
                n3417 = case shown="1..10, Default" w4689 {
                  tunnel: [1 3] -> w4696
                  frame 1..10, Default {
                  }
                  frame 11.. {
                  }
                }
                n3418 = case shown="0..10, Default" w4688 {
                  tunnel: [1 2 3] -> w4695
                  frame 0..10, Default {
                  }
                  frame 11, 12 {
                  }
                  frame 13.. {
                  }
                }
                n3419 = case shown="3601.." w4691 {
                  tunnel: [1 2 3] -> w4690
                  frame 0..3000, Default {
                    # "Normal"
                  }
                  frame 3001..3600 {
                  }
                  frame 3601.. {
                  }
                }
                n3420 = Or(x=w4668, y=w4667) -> (x .or. y?=w4666:bool)
                n3421 = Greater Or Equal?(x=w4671, y=w4655) -> (x >= y?=w4658:bool)
                n3422 = case shown="0, 1, Default" w4671 {
                  tunnel: [1 3] -> w4654
                  frame 0, 1, Default {
                  }
                  frame 2.. {
                  }
                }
                n3423 = case shown="True" w4658 {
                  tunnel: [1 3] -> w4653
                  frame False {
                  }
                  frame True {
                  }
                }
                n3424 = case shown="True" w4666 {
                  tunnel: [1 2] -> w4652
                  frame False {
                  }
                  frame True {
                  }
                }
                n3425 = Build Array(w4678, w4677, w4676) -> (w4675:i32[])
                n3426 = Number To Decimal String(number=w4690) -> (decimal integer string=→"sp_st":string)  [unwired: 1 in]
                n3427 = Array Max & Min(array=w4675) -> (max value=w4672:i32)  [unwired: 3 out]
                "TEMP STATE" <- w4672
                n3428 = Number To Decimal String(number=w4696) -> (decimal integer string=w4699:string)  [unwired: 1 in]
                n3429 = Number To Decimal String(number=w4695) -> (decimal integer string=w4697:string)  [unwired: 1 in]
                n3430 = Number To Decimal String(number=w4672) -> (decimal integer string=→"temp_st":string)  [unwired: 1 in]
                n3431 = Build Array(w4654, w4653, w4652) -> (w4651:i32[])
                n3432 = local write "nl_st"(w4699) -> ()
                n3433 = local write "ff_st"(w4697) -> ()
                n3434 = Number To Decimal String(number=1) -> (decimal integer string=w4694:string)  [unwired: 1 in]
                n3435 = Array Max & Min(array=w4651) -> (max value=w4650:i32)  [unwired: 3 out]
                n3436 = local write "Air temp"(w4694) -> ()
                n3437 = Number To Decimal String(number=w4650) -> (decimal integer string=w4649:string)  [unwired: 1 in]
                n3438 = local write "Stroke Ln 2"(w4649) -> ()
              }
            }
            n3439 = local read "Stroke Ln 2"() -> (w4561:string)
            n3440 = local read "nl_st"() -> (w4567:string)
            n3441 = local read "ff_st"() -> (w4564:string)
            n3442 = local read "sp_st"() -> (w4565:string)
            n3443 = local read "temp_st"() -> (w4566:string)
            n3444 = local read "Air temp"() -> (w4560:string)
            n3445 = Replace Array Subset(array="in", new element #1=w4567, index #1=1 ("index"), new element #2=w4564, index #2=2 ("index"), new element #3=w4566, index #3=3 ("index"), new element #4=w4565, index #4=4 ("index"), new element #5=w4561, index #5=5 ("index"), new element #6=w4560, index #6=6 ("index"), new element #7="Sensor State" ("new element/subarray"), index #7=0 ("index")) -> (→"out":string[])
          }
        }
        n3446 = Wait (ms)(milliseconds to wait=u32 10) -> ()  [unwired: 1 out]
        n3447 = local read "Quit"() -> (w4555:bool)
      }
      n3448 = while {
        stop <- w4530 stop-if-true
        n3449 = local read "run replace"() -> (w4532:bool)
        n3450 = Wait (ms)(milliseconds to wait=u32 100) -> ()  [unwired: 1 out]
        n3451 = Equal?(x="FLAG 2", y=0.0) -> (x = y?=w4533:bool)
        n3452 = case shown="True" w4533 {
          frame False {
          }
          frame True {
            n3453 = local write "FLAG 2"(100.0 ("FLAG 2")) -> ()
            n3454 = call <vilib>:"Read Characters From File.vi"("file path (dialog if empty)"=path "C:/LAB-IQ-NXT/WO 2449 TT.sig", "convert eol? (no:F)"=FALSE ("append to file? (new file:F)")) -> ("character string"=w4536:string)  [unwired: 4 in, 3 out]
            n3455 = call <vilib>:"Read Characters From File.vi"("file path (dialog if empty)"=path "C:/LAB-IQ-NXT/WO 2449 TRH.sig", "convert eol? (no:F)"=FALSE ("append to file? (new file:F)")) -> ("character string"=w4537:string)  [unwired: 4 in, 3 out]
            n3456 = Decimal String To Number(string=w4536) -> (number=w4538:i32)  [unwired: 2 in, 1 out]
            n3457 = local write "Total No. of Tests"(w4538) -> ()
            n3458 = Decimal String To Number(string=w4537) -> (number=w4541:i32)  [unwired: 2 in, 1 out]
            n3459 = local write "SEN.RUN HRS"(w4541) -> ()
          }
        }
        n3460 = case shown="True" w4532 {
          frame False {
          }
          frame True {
            n3461 = Equal?(x="FLAG 4", y=0.0) -> (x = y?=w4545:bool)
            n3462 = case shown="False" w4545 {
              frame False {
                n3463 = Get Date/Time In Seconds() -> (seconds since 1Jan1904=w4551:timestamp)
                n3464 = local read "START 3"() -> (w4549:dbl)
                n3465 = To Double Precision Float(number=w4551) -> (double precision float=w4550:dbl)
                n3466 = Subtract(x=w4550, y=w4549) -> (x-y=→"SENSOR TIME":dbl)
              }
              frame True {
                n3467 = Get Date/Time In Seconds() -> (seconds since 1Jan1904=w4553:timestamp)
                n3468 = local write "FLAG 4"(100.0 ("FLAG")) -> ()
                n3469 = To Double Precision Float(number=w4553) -> (double precision float=→"START 3":dbl)
              }
            }
          }
        }
        n3470 = local read "Quit"() -> (w4530:bool)
      }
      n3471 = while {
        shift-right: [w4330] -> _
        shift-left: _ -> [w4331]
        tunnel: [w4326] -> _
        i -> [w4326]
        stop <- w4325 stop-if-true
        n3472 = Wait (ms)(milliseconds to wait=u32 50 ("Refresh Rate (ms)")) -> ()  [unwired: 1 out]
        n3473 = local read "Json End Flg"() -> (w4327:bool)
        n3474 = Not(x="Upld AR 2") -> ()  [unwired: 1 out]
        n3475 = local read "Upld AR 2"() -> (w4328:bool)
        n3476 = call "Elapsed Time9"("Time Target (s)"="Sen.Upload Rate (s)", "Reset"=FALSE, "Auto Reset"=TRUE) -> ("Time has Elapsed"=w4337:bool)  [unwired: 9 in, 7 out]
        n3477 = Or(x=w4337, y=w4327) -> (x .or. y?=w4333:bool)
        n3478 = case shown="True" w4333 {
          frame False {
          }
          frame True {
            w4429 = "\"SensorName\":\"" ("string")
            w4399 = " \"},{"
            w4424 = "\",\"SensorState\":\""
            w4426 = "\",\"SensorModelNumber\":\"" ("string")
            w4425 = "\",\"SensorRuntimeHours\":\"" ("string")
            n3479 = local read "model num"() -> (w4423:string[])
            n3480 = local read "Sensor name"() -> (w4442:string[])
            n3481 = local read "run"() -> (w4413:string[])
            n3482 = local read "SENSOR TIME"() -> (w4369:dbl)
            n3483 = local read "out"() -> (w4362:string[])
            n3484 = local read "Total No. of Tests"() -> (w4367:dbl)
            n3485 = Select(t=60.0, s="Run test 3", f=3600.0) -> (s? t:f=w4377:dbl)
            n3486 = Index Array(array=w4423, index #1=1 ("index")) -> (element #1=w4422:string, element #2=w4421:string, element #3=w4420:string, element #4=w4419:string, element #5=w4418:string, element #6=w4417:string)  [unwired: 5 in]
            n3487 = Index Array(array=w4413, index #1=1 ("index")) -> (element #1=w4412:string, element #2=w4411:string, element #3=w4410:string, element #4=w4409:string, element #5=w4408:string, element #6=w4407:string)  [unwired: 5 in]
            n3488 = Index Array(array=w4442, index #1=1 ("index")) -> (element #1=w4441:string, element #2=w4440:string, element #3=w4439:string, element #4=w4438:string, element #5=w4428:string, element #6=w4427:string)  [unwired: 5 in]
            n3489 = Index Array(array=w4362, index #1=1 ("index")) -> (element #1=w4394:string, element #2=w4393:string, element #3=w4392:string, element #4=w4391:string, element #5=w4390:string, element #6=w4389:string)  [unwired: 5 in]
            n3490 = local read "SEN.RUN HRS"() -> (w4365:dbl)
            n3491 = Divide(x=w4369, y=w4377) -> (x/y=w4376:dbl)
            n3492 = Increment(x=w4376) -> (x+1=w4372:dbl)
            n3493 = Number To Decimal String(number=w4372) -> (decimal integer string=→"run hrs":string)  [unwired: 1 in]
            n3494 = Divide(x=w4365, y=3600.0 ("f")) -> (x/y=w4360:dbl)
            n3495 = Round To Nearest(number=w4360) -> (nearest integer value=w4358:dbl)
            n3496 = Number To Decimal String(number=w4358) -> (decimal integer string=w4359:string)  [unwired: 1 in]
            n3497 = Number To Decimal String(number=w4367) -> (decimal integer string=w4368:string)  [unwired: 1 in]
            n3498 = local read "Model No"() -> (w4373:string)
            n3499 = local read "UUID"() -> (w4468:string)
            n3500 = local read "Serial No"() -> (w4472:string)
            n3501 = local read "Secret Key"() -> (w4473:string)
            n3502 = Concatenate Strings("\",\"MachineSerialNumber\":\"" ("string"), w4472) -> (w4476:string)
            n3503 = Concatenate Strings("\",\"ModelNumber\":\"" ("string"), w4373) -> (w4374:string)
            n3504 = Concatenate Strings("\",\"MachineRuntimeHours\":\"" ("string"), w4359) -> (w4477:string)
            n3505 = Concatenate Strings("\",\"MachineRuntimeCycles\":\"", w4368) -> (w4470:string)
            n3506 = Concatenate Strings(w4426, w4422) -> (w4456:string)
            n3507 = Concatenate Strings(w4425, w4412) -> (w4457:string)
            n3508 = Concatenate Strings(w4424, w4394) -> (w4455:string)
            n3509 = Concatenate Strings(w4476, w4374, w4477, w4470) -> (w4479:string)
            n3510 = Concatenate Strings(w4426, w4421) -> (w4453:string)
            n3511 = Concatenate Strings(w4425, w4411) -> (w4452:string)
            n3512 = Concatenate Strings(w4424, w4393) -> (w4454:string)
            n3513 = Concatenate Strings(w4426, w4420) -> (w4448:string)
            n3514 = Concatenate Strings(w4425, w4410) -> (w4449:string)
            n3515 = Concatenate Strings(w4424, w4392) -> (w4447:string)
            n3516 = Concatenate Strings(w4426, w4419) -> (w4445:string)
            n3517 = Concatenate Strings(w4425, w4409) -> (w4444:string)
            n3518 = Concatenate Strings(w4424, w4391) -> (w4446:string)
            n3519 = Concatenate Strings(w4456, w4457, w4455) -> (w4458:string)
            n3520 = Concatenate Strings(w4426, w4418) -> (w4435:string)
            n3521 = Concatenate Strings(w4425, w4408) -> (w4436:string)
            n3522 = Concatenate Strings(w4426, w4417) -> (w4432:string)
            n3523 = Concatenate Strings(w4425, w4407) -> (w4431:string)
            n3524 = Concatenate Strings(w4424, w4390) -> (w4434:string)
            n3525 = Concatenate Strings(w4424, w4389) -> (w4433:string)
            n3526 = Concatenate Strings("{\"SecretKey\":\"", w4473, w4479, "\",\"UUID\" : \"", w4468, "\",\"SensorInformation\":", "[{" ("string")) -> (w4406:string)
            n3527 = Concatenate Strings(w4453, w4452, w4454) -> (w4451:string)
            n3528 = Concatenate Strings(w4448, w4449, w4447) -> (w4450:string)
            n3529 = Concatenate Strings(w4445, w4444, w4446) -> (w4443:string)
            n3530 = Concatenate Strings(w4435, w4436, w4434) -> (w4437:string)
            n3531 = Concatenate Strings(w4432, w4431, w4433) -> (w4430:string)
            n3532 = Concatenate Strings(w4429, w4441, w4458, w4399) -> (w4405:string)
            n3533 = Concatenate Strings(w4429, w4440, w4451, w4399) -> (w4404:string)
            n3534 = Concatenate Strings(w4429, w4439, w4450, w4399) -> (w4403:string)
            n3535 = Concatenate Strings(w4429, w4438, w4443, w4399) -> (w4402:string)
            n3536 = Concatenate Strings(w4429, w4428, w4437, w4399) -> (w4401:string)
            n3537 = Concatenate Strings(w4429, w4427, w4430, "\"}" ("string")) -> (w4400:string)
            n3538 = Concatenate Strings(w4406, w4405, w4404, w4403, w4402, w4401, w4400, "]}" ("string")) -> (w4397:string)
            n3539 = local read "SEN.RUN HRS"() -> (w4364:dbl)
            n3540 = disable-structure shown="Disabled" {
              frame Disabled {
                n3541 = local read "state"() -> (w4483:string[])
                n3542 = Delete From Array(array=w4483, index=0) -> (array with subset deleted=w4481:string[])  [unwired: 1 in, 1 out]
                n3543 = for {
                  N: 6 -> [_]
                  tunnel: w4481 -> [w4494] mode=indexing
                  tunnel: [w4493] -> w4480 mode=indexing
                  n3544 = Equal?(x=w4494, y="Warning") -> (x = y?=w4490:bool)
                  n3545 = Equal?(x=w4494, y="Healthy") -> (x = y?=w4487:bool)
                  n3546 = Select(t="2" ("y"), s=w4490, f="3" ("y")) -> (s? t:f=w4485:string)
                  n3547 = Select(t="1" ("y"), s=w4487, f=w4485) -> (s? t:f=w4493:string)
                }
                "state1" <- w4480
              }
              frame Enabled {
              }
            }
            n3548 = stacked-sequence {
              tunnel: w4397 -> [w4505 _ _]
              tunnel: [_ _ w4521] -> _
              frame #0 {
                (unwired) FALSE ("convert eol (F)")
                w4507 = enum16{"start", "end", "current"}."start" ("pos mode (0:2)")
                n3549 = local read "Path"() -> (w4501:path)
                n3550 = Path To String(path=w4501) -> (string=w4513:string)
                n3551 = Concatenate Strings(w4513, "\\", "Sensor File Name") -> (w4514:string)
                n3552 = local write "standard output 2"(" ") -> ()
                n3553 = String To Path(string=w4514) -> (path=w4504:path)
                n3554 = call <vilib>:"Open_Create_Replace File.vi"("advisory dialog? (display:T)"=FALSE, "function (open:0)"=T27."create or replace", "file path"=w4504) -> ("error out"=w4517:errorcluster, "refnum"=w4516:refnum<file>)  [unwired: 5 in, 2 out]
                n3555 = Set File Position(refnum=w4516, from (0:start)=w4507, error in=w4517) -> (refnum out=w4497:refnum<file>, error out=w4496:errorcluster)  [unwired: 1 in]
                n3556 = Write to Binary File(file (use dialog)=w4497, data=" ", error in=w4496, 5:FALSE ("prepend array or string size? (T)")) -> (refnum out=w4508:refnum<file>, error out=w4509:errorcluster)  [unwired: 2 in, 1 out]
                n3557 = Set File Position(offset (in bytes) (0)=w4507, refnum=w4508, error in=w4509) -> (refnum out=w4500:refnum<file>, error out=w4499:errorcluster)  [unwired: 1 in]
                n3558 = Write to Binary File(file (use dialog)=w4500, data=w4505, error in=w4499, 5:FALSE ("prepend array or string size? (T)")) -> (error out=w4503:errorcluster)  [unwired: 2 in, 2 out]
                n3559 = flat-sequence {
                  tunnel: w4504 -> [w4519]
                  tunnel: w4503 -> [_]
                  frame #0 {
                    n3560 = call <vilib>:"Read Characters From File.vi"("file path (dialog if empty)"=w4519) -> ("character string"=→"Sensor Health JSON string":string)  [unwired: 5 in, 3 out]
                  }
                }
                "SinglePoint  2" <- w4505
              }
              frame #1 {
              }
              frame #2 {
                (unwired) "\"Stored\": true" ("string")
                n3561 = call <vilib>:"System Exec.vi"("run minimized? (F)"=TRUE, "wait until completion? (T)"=TRUE, "working directory"=path "C:/LAB-IQ-NXT", "command line"="C:\\LAB-IQ-NXT\\JPostH.bat") -> ("standard error"=→"Respose From Server 2":string, "standard output"=w4524:string)  [unwired: 4 in, 2 out]
                "standard output 2" <- w4524
                n3562 = Match Pattern(string=w4524, regular expression="JSONH Check String") -> (match substring=w4522:string, offset past match=w4521:i32)  [unwired: 1 in, 2 out]
                n3563 = Equal?(x=w4522, y="JSONH Check String") -> (x = y?=→"Upload \nConfirmed 2":bool)
              }
            }
            n3564 = Divide(x=w4364, y=3600.0 ("f")) -> (x/y=w4357:dbl)
            n3565 = local read "run time"() -> (w4414:string[])
            n3566 = Round To Nearest(number=w4357) -> (nearest integer value=w4356:dbl)
            n3567 = Number To Decimal String(number=w4356) -> (decimal integer string=w4355:string)  [unwired: 1 in]
            n3568 = Index Array(array="Sensor Information", index (col) #1=0 ("disabled index (col)"), index (col) #2=1 ("index (col)"), index (col) #3=2 ("index (col)"), index (col) #4=3 ("index (col)")) -> (element #1=→"Sensor name":string[], element #2=→"model num":string[], element #3=→"run time":string[], element #4=→"state":string[])  [unwired: 4 in]
            n3569 = Insert Into Array(array=w4414, index=1, new element #1=w4355, new element #2=w4355, new element #3=w4355, new element #4=w4355, new element #5=w4355, new element #6=w4355) -> (w4379:string[])
            "run" <- w4379
            n3570 = local read "out"() -> (w4361:string[])
            n3571 = local read "Sensor Information"() -> (w4381:string[][])
            n3572 = Replace Array Subset(array=w4381, new element #1=w4379, index (col) #1=2 ("disabled index (col)"), new element #2=w4361, index (col) #2=3 ("index (col)")) -> (w4380:string[][])  [unwired: 2 in]
            n3573 = local write "Sensor Information"(w4380) -> ()
          }
        }
        n3574 = case shown="True" w4328 {
          frame False {
          }
          frame True {
            n3575 = Equal?(x="FLAG", y=0.0) -> (x = y?=w4345:bool)
            n3576 = case shown="False" w4345 {
              frame False {
                n3577 = Get Date/Time In Seconds() -> (seconds since 1Jan1904=w4351:timestamp)
                n3578 = local read "START 2"() -> (w4349:dbl)
                n3579 = To Double Precision Float(number=w4351) -> (double precision float=w4350:dbl)
                n3580 = Subtract(x=w4350, y=w4349) -> (x-y=→"SENSOR TIME  2":dbl)
              }
              frame True {
                n3581 = Get Date/Time In Seconds() -> (seconds since 1Jan1904=w4353:timestamp)
                n3582 = To Double Precision Float(number=w4353) -> (double precision float=→"START 2":dbl)
                n3583 = local write "FLAG"(100.0 ("FLAG")) -> ()
              }
            }
          }
        }
        n3584 = disable-structure shown="Disabled" {
          disable-tunnel: w4331 -> [w4340 _]
          disable-tunnel: [w4339 _] -> w4330
          frame Disabled {
            n3585 = local read "Json St Flg"() -> (w4338:bool)
            n3586 = case shown="True" w4338 {
              tunnel: w4340 -> [w4341 w4343]
              tunnel: [w4341 w4342] -> w4339
              frame False {
              }
              frame True {
                n3587 = Increment(x=w4343) -> (x+1=w4342:dbl)
                "T cycle" <- w4342
                n3588 = local write "Json St Flg"(FALSE ("Json St Flg")) -> ()
